vi "mupExpr Multi Test.vi"() -> ()   [LabVIEW 2015]
uses:
  mupExpr/mupExpr.lvclass/mupExpr.ctl
  mupExpr/SetVarVal.vi
  mupLib/mupEval.vi
  mupLib/mupSetVarValue.vi
  mupLib/mupCheckError.vi
  mupLib/mupLibPath.vi
  <vilib>/Utility/error.llb/Error Cluster From Error Code.vi
  mupExpr/mupExpr.lvclass
panel:
  out "Array":dbl[][](array[numeric])
  out "Instance":i32
  out "Result":dbl
  out "error out":errorcluster
  in  "Instances":i32=10
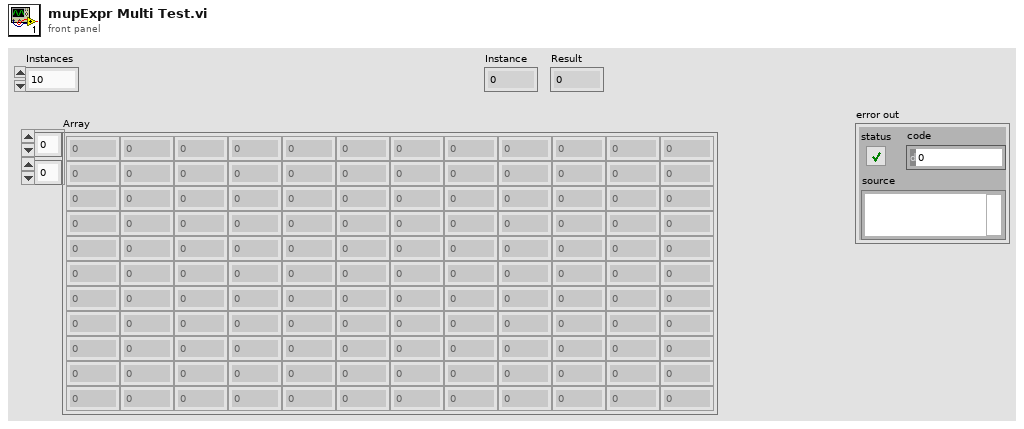
[diagram p1: front panel]
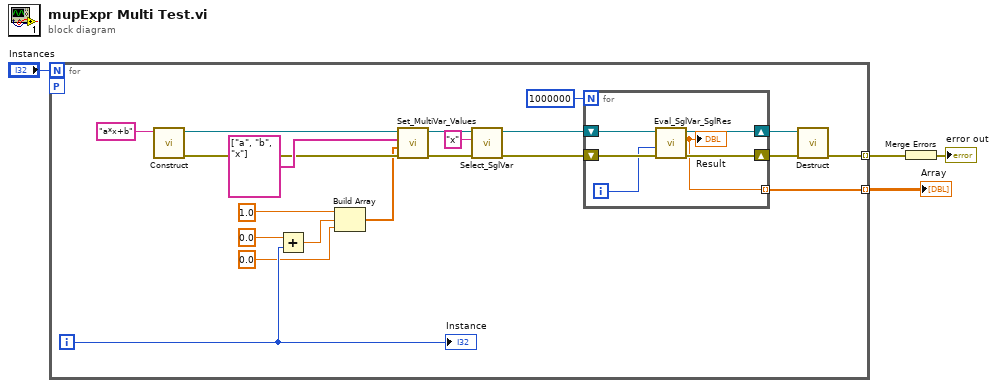
[diagram p0: block diagram]
diagram:
  n1 = for {
    N: "Instances" -> [_]
    tunnel: [w6] -> w2 mode=indexing
    workers-P: _ -> [_]
    tunnel: [w5] -> w1 mode=indexing
    i -> [w19]
    n2 = call "Construct.vi"("Expression"="a*x+b") -> ("error out"=w21:errorcluster, "mupExpr out"=w23:refnum<data-value>)  [unwired: 8 in, 1 out]
    n3 = Add(x=0.0, y=w19) -> (x+y=w17:dbl)
    n4 = Build Array(1.0, w17, 0.0) -> (w15:dbl[])
    n5 = call "Set_MultiVar_Values.vi"("error in (no error)"=w21, "varValues"=w15, "varNames"=string[] ["a", "b", "x"], "mupExpr in"=w23) -> ("error out"=w13:errorcluster, "mupExpr out"=w14:refnum<data-value>)  [unwired: 6 in]
    n6 = call "Select_SglVar.vi"("error in (no error)"=w13, "varName"="x", "mupExpr in"=w14) -> ("error out"=w9:errorcluster, "mupExpr out"=w10:refnum<data-value>)  [unwired: 7 in]
    n7 = for {
      N: 1000000 -> [_]
      shift-right: [w27] -> w8
      shift-left: w10 -> [w30]
      shift-right: [w28] -> w7
      shift-left: w9 -> [w29]
      tunnel: [w25] -> w5 mode=indexing
      i -> [w26]
      n8 = call "Eval_SglVar_SglRes.vi"("error in (no error)"=w29, "varValue"=w26, "mupExpr in"=w30) -> ("error out"=w28:errorcluster, "Result"=w25:dbl, "mupExpr out"=w27:refnum<data-value>)  [unwired: 6 in]
      "Result" <- w25
    }
    n9 = call "Destruct.vi"("error in (no error)"=w7, "mupExpr in"=w8) -> ("error out"=w6:errorcluster)  [unwired: 9 in]
    "Instance" <- w19
  }
  "Array" <- w1
  n10 = Merge Errors(w2) -> (→"error out":errorcluster)
